vi "Progress.vi"(8 "error in":errorcluster, 11 "UserInterface in":refnum<class "UserInterface.lvclass">) -> (0 "error out":errorcluster, 3 "UserInterface out":refnum<class "UserInterface.lvclass">)   [LabVIEW 2021, in "UserInterface.lvlib" / "UserInterface.lvclass"]
uses:
  UserInterface.lvclass
  UserInterface.lvclass/UserInterface.ctl
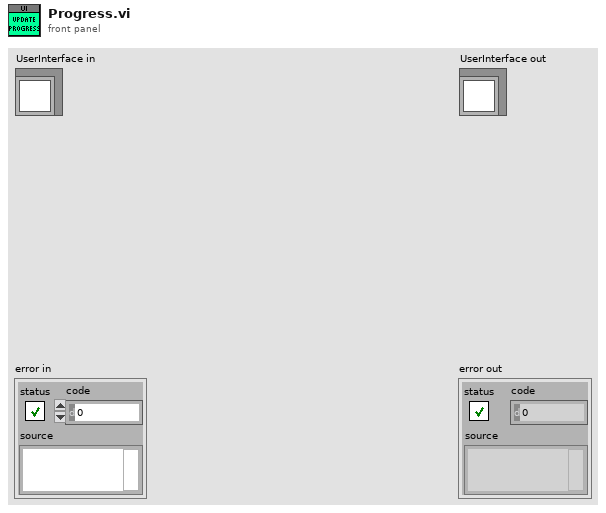
[diagram p1: front panel]
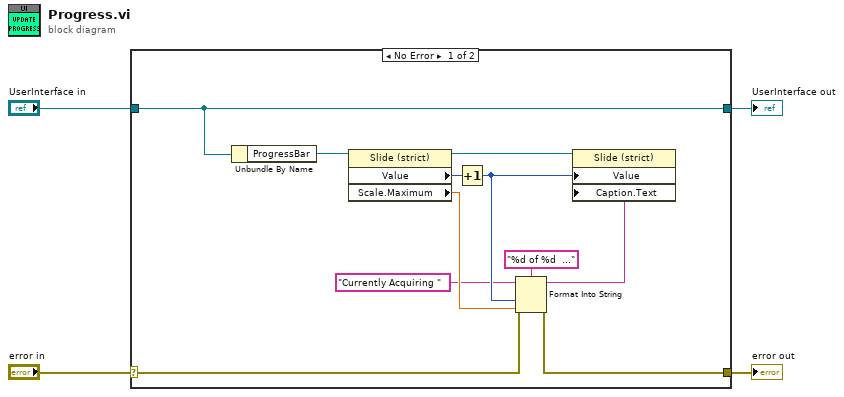
[diagram p0: block diagram]
diagram:
  n1 = case shown="No Error" "error in" {
    selector: "error in" -> [w6 w17]
    tunnel: [w5 w17] -> w3
    tunnel: [w15 w16] -> w1
    tunnel: "UserInterface in" -> [w15 w16]
    frame No Error {
      n2 = Unbundle By Name(w15) -> ("ProgressBar"=w14:refnum<vi>)
      n3 = property class="Slide (strict)"(reference=w14) -> (reference out=w12:refnum<vi>, "Value"=w13:u32, "Scale.Maximum"=w11:dbl)  [unwired: 1 in, 1 out]
      n4 = Increment(x=w13) -> (x+1=w10:u32)
      n5 = Format Into String(format string="%d of %d  ...", initial string="Currently Acquiring ", error in=w6, w10, w11) -> (resulting string=w7:string, error out=w5:errorcluster)
      n6 = property class="Slide (strict)"(reference=w12, "Value"=w10, "Caption.Text"=w7) -> ()  [unwired: 1 in, 2 out]
    }
    frame Error {
    }
  }
  "error out" <- w3
  "UserInterface out" <- w1
